vi "LV SciSDK OSCILLOSCOPE DUAL.vi"(7 "Oscilloscope Dual Handle In":T3, 9 "Board Handle In":T1, 11 "error in (no error)":errorcluster) -> (4 "NI Error Code":i64, 6 "Oscilloscope Dual Buffer Out":T2, 8 "Oscilloscope Dual Handle Out":T3, 10 "Board Handle Out":T1, 15 "error out":errorcluster)   [LabVIEW 2021, in "SciSDK_Labview.lvlib"]
uses:
  SciSDK_Labview.lvlib
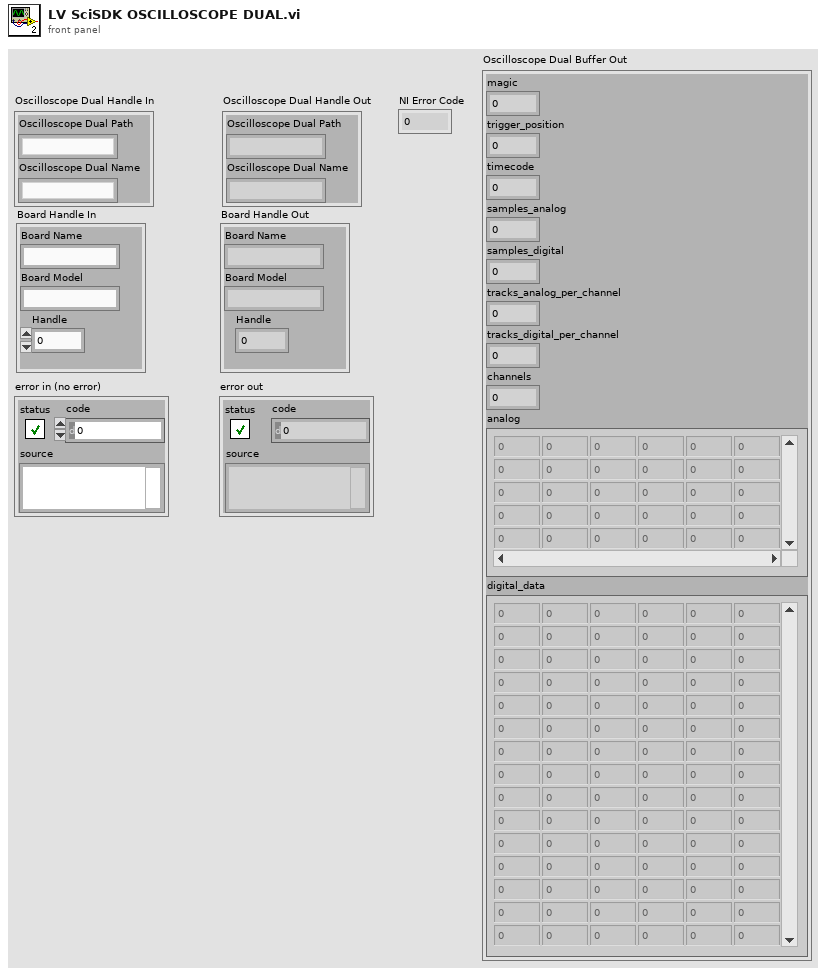
[diagram p1: front panel]
types:
  T1 = cluster{"Board Name":string, "Board Model":string, "Handle":u64}
  T2 = cluster{"magic":u32, "trigger_position":u32, "timecode":u32, "samples_analog":u32, "samples_digital":u32, "tracks_analog_per_channel":u32, "tracks_digital_per_channel":u32, "channels":u32, "analog":dbl[][], "digital_data":i32[][]}
  T3 = cluster{"Oscilloscope Dual Path":string, "Oscilloscope Dual Name":string}
  T4 = cluster{"magic":u32, "trigger_position":u32, "timecode":u32, "samples_analog":u32, "samples_digital":u32, "tracks_analog_per_channel":u32, "tracks_digital_per_channel":u32, "channels":u32, "analog":i32[][], "digital_data":i32[][]}
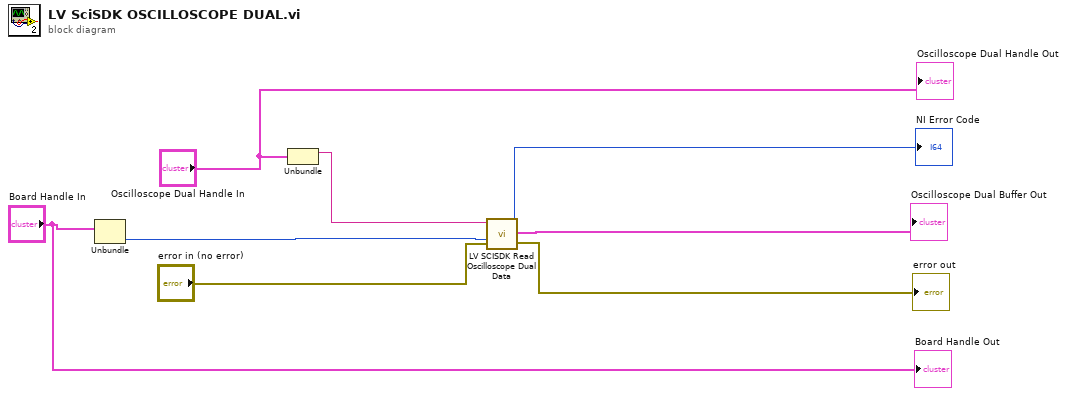
[diagram p0: block diagram]
diagram:
  n1 = Unbundle("Board Handle In") -> ("Handle"=w1:u64)  [unwired: 2 out]
  n2 = Unbundle("Oscilloscope Dual Handle In") -> ("Oscilloscope Dual Path"=w3:string)  [unwired: 1 out]
  n3 = call "LV SCISDK Read Oscilloscope Dual Data.vi"("Path"=w3, "handle"=w1, "error in (no error)"="error in (no error)") -> ("function return"=→"NI Error Code":i32, "buffer out"=→"Oscilloscope Dual Buffer Out":T4, "error out"=→"error out":errorcluster)  [unwired: 4 in, 1 out]
  "Oscilloscope Dual Handle Out" <- "Oscilloscope Dual Handle In"
  "Board Handle Out" <- "Board Handle In"
